vi "Acquire.vi"(8 "error in (no error)":errorcluster, 9 "piint (readout_time_out)":i64, 10 "readout_count":i64, 11 "camera handle in":u64) -> (0 "error out":errorcluster, 3 "camera handle out":u64)   [LabVIEW 2019, in "PICam.lvlib"]
doc: "Picam_Acquire() performs a specified number of data readouts (specified by readout_count) and returns once the acquisition has been completed.\n\nThis function cannot be called when hardware is configured for non-destructive readout. This is because the number of readouts acquired is no longer guaranteed to be fixed. As an example, changing the exposure time online will change the number of non-destructive readouts and therefore the total number of readouts acquired.\n\nParameters must be committed prior to initiating data acquisition. Refer to Section 5.4.6.2, Picam_CommitParameters(), on page 177 for additional information."
uses:
  PICam.lvlib
  types/PicamAvailableData.ctl
  Picam64.dll
panel:
  out "PicamAvailableData* (available)":T1
  out "PicamAcquisitionErrorsMask* (errors)":u64
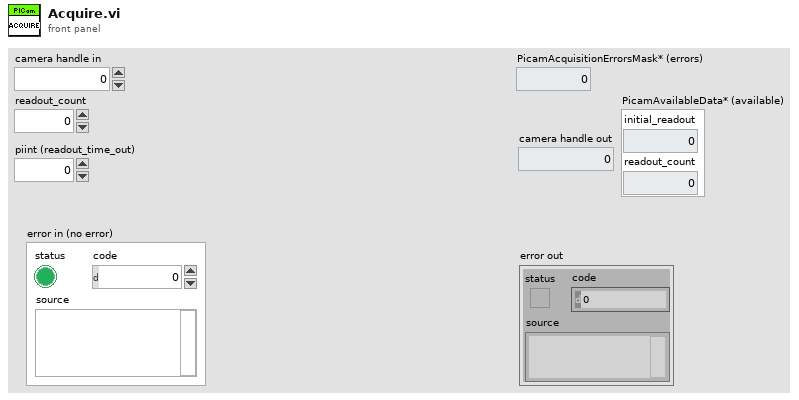
[diagram p1: front panel]
types:
  T1 = typedef "PicamAvailableData.ctl" = cluster{"initial_readout":u64, "readout_count":i64}
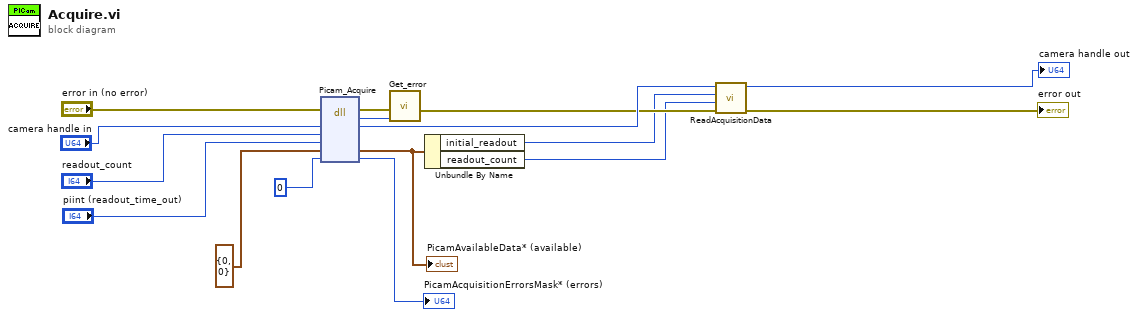
[diagram p0: block diagram]
diagram:
  n1 = dll-call lib="Picam*.*" fn="Picam_Acquire"(error in="error in (no error)", "PicamHandle (camera)"="camera handle in", "pi64s (readout_count)"="readout_count", "piint (readout_time_out)"="piint (readout_time_out)", "PicamAvailableData* (available)"=T1 {"initial_readout"=0, "readout_count"=0} ("PicamAvailableData"), "PicamAcquisitionErrorsMask* (errors)"=u8 0) -> (error out=w15:errorcluster, "err"=w16:u64, "PicamHandle (camera)"=w7:u64, "PicamAvailableData* (available)"=w3:T1, "PicamAcquisitionErrorsMask* (errors)"=→"PicamAcquisitionErrorsMask* (errors)":u8)  [unwired: 4 in, 1 out]
  "PicamAvailableData* (available)" <- w3
  n2 = call "Get_error.vi"("PICam_Error"=w16, "error in (no error)"=w15) -> ("error out"=w6:errorcluster)  [unwired: 9 in]
  n3 = Unbundle By Name(w3) -> ("initial_readout"=w2:u64, "readout_count"=w1:i64)
  n4 = call "ReadAcquisitionData.vi"("error in (no error)"=w6, "readout_count"=w1, "initial_readout*"=w2, "PicamHandle (camera)"=w7) -> ("error out"=→"error out":errorcluster, "camera handle out"=→"camera handle out":i64)  [unwired: 6 in]
